vi "Configure Temperature Units.vi"(5 "Retry Attempts (0)":i32 min=0, 7 "Unit Address (-1)":i32=-1, 8 "error in (no error)":errorcluster, 10 "Temperature Units (Celsius)":T1=enum."Celsius", 11 "VISA resource name (in)":refnum<visa-resource-name>) -> (0 "error out":errorcluster, 2 "Response Cluster":T2 {"Command ID" format="%x"}, 3 "VISA resource name (out)":refnum<visa-resource-name>)   [LabVIEW 2020, in "Omega Platinum Series.lvlib"]
doc: "Change the temperature units the unit converts to."
uses:
  Omega Platinum Series.lvlib
  Type Defs/Response.ctl
  Type Defs/Display Temperature Units.ctl
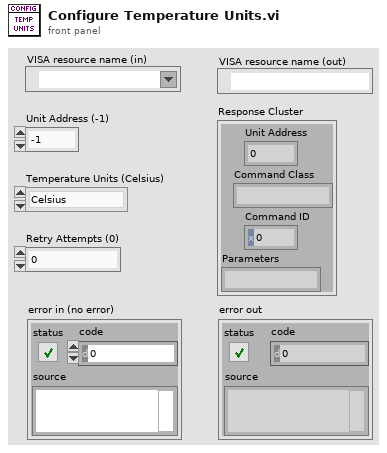
[diagram p1: front panel]
types:
  T1 = typedef "Omega Platinum Series.lvlib/Display Temperature Units.ctl" = enum16{"No units applied", "Celsius", "Fahrenheit"}
  T2 = typedef "Omega Platinum Series.lvlib/Response.ctl" = cluster{"Unit Address":i32, "Command Class":string, "Command ID":u32, "Parameters":string}
  T3 = typedef "Omega Platinum Series.lvlib/Display Decimal Point.ctl" = enum16{"F.FFF", "FF.FF"}
  T4 = typedef "Omega Platinum Series.lvlib/Display Color.ctl" = enum16{"GREEN", "RED", "AMBER"}
  T5 = typedef "Omega Platinum Series.lvlib/Display Brightness.ctl" = enum16{"LOW", "MEDIUM", "HIGH"}
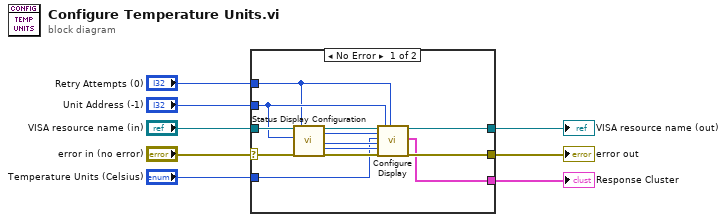
[diagram p0: block diagram]
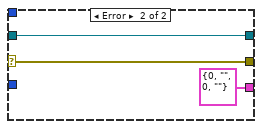
[diagram p2: hidden frame]
diagram:
  n1 = case shown="No Error" "error in (no error)" {
    selector: "error in (no error)" -> [w21 w24]
    tunnel: "Temperature Units (Celsius)" -> [w12 _]
    tunnel: "Unit Address (-1)" -> [w16 _]
    tunnel: [w19 w24] -> w6
    tunnel: "VISA resource name (in)" -> [w18 w23]
    tunnel: [w10 w23] -> w4
    tunnel: [w11 T2 {"Unit Address"=0, "Command Class"="", "Command ID"=0, "Parameters"=""} ("Response Cluster")] -> w3
    tunnel: "Retry Attempts (0)" -> [w9 _]
    frame No Error {
      n2 = call "Status Display Configuration.vi"("VISA resource name (in)"=w18, "Unit Address (-1)"=w16, "error in (no error)"=w21, "Retry Attempts (0)"=w9) -> ("VISA resource name (out)"=w17:refnum<visa-resource-name>, "Decimal Point"=w15:T3, "Display Color"=w14:T4, "Display Brightness"=w13:T5, "error out"=w20:errorcluster)  [unwired: 10 in, 1 out]
      n3 = call "Configure Display.vi"("VISA resource name (in)"=w17, "Decimal Point (F.FFF)"=w15, "Temperature Units (none)"=w12, "Display Color (GREEN)"=w14, "Display Brightness (LOW)"=w13, "error in (no error)"=w20, "Unit Address (-1)"=w16, "Retry Attempts (0)"=w9) -> ("VISA resource name (out)"=w10:refnum<visa-resource-name>, "Response Cluster"=w11:T2, "error out"=w19:errorcluster)  [unwired: 9 in]
    }
    frame Error {
    }
  }
  "error out" <- w6
  "VISA resource name (out)" <- w4
  "Response Cluster" <- w3
